vi "py-lv-comm_closeConnection.vi"(8 "error in (no error)":errorcluster, 10 "socket in":refnum<class "zmq_socket.lvclass">, 11 "zmq_context in":refnum<class "zmq_context.lvclass">) -> (0 "error out":errorcluster)   [LabVIEW 2016]
uses:
  <vilib>/addons/zeromq/zmq_socket.lvclass
  <vilib>/addons/zeromq/zmq_context.lvclass
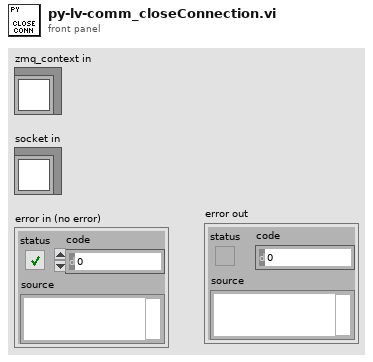
[diagram p1: front panel]
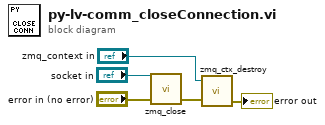
[diagram p0: block diagram]
diagram:
  n1 = call <vilib>:"zmq_close.vi"("error in"="error in (no error)", "socket"="socket in") -> ("error out"=w3:errorcluster)  [unwired: 3 in]
  n2 = call <vilib>:"zmq_ctx_destroy.vi"("error in"=w3, "context in"="zmq_context in") -> ("error out"=→"error out":errorcluster)  [unwired: 3 in]
